vi "expressVI.vi"() -> ()   [LabVIEW 2020]
uses:
  <vilib>/express/express arith-compare/Formula/XNode/ExpressFormulaBlockNode.xnode
panel:
  out "数值":dbl=2.0
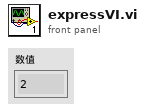
[diagram p1: front panel]
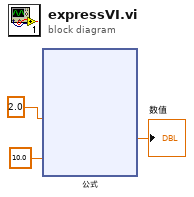
[diagram p0: block diagram]
diagram:
  n1 = xnode "公式"("X1"=2.0, "X2"=10.0) -> ("结果"=→"数值":dbl)  [unwired: 1 in, 1 out]
